vi "Test Null Assert.vi"(7 "Label (VI Title)":string, 8 "error in (no error)":errorcluster, 10 "Type in":variant, 11 "Type in":variant) -> (0 "error out":errorcluster)   [LabVIEW 2018, in "JSON to LVConstant Test.lvlib"]
uses:
  JSON to LVConstant Test.lvlib
  <vilib>/addons/_JKI Toolkits/Caraya/classes/Assert/Assert True.vi
  <vilib>/addons/_JKI Toolkits/Caraya/classes/Assert/Assert.lvclass
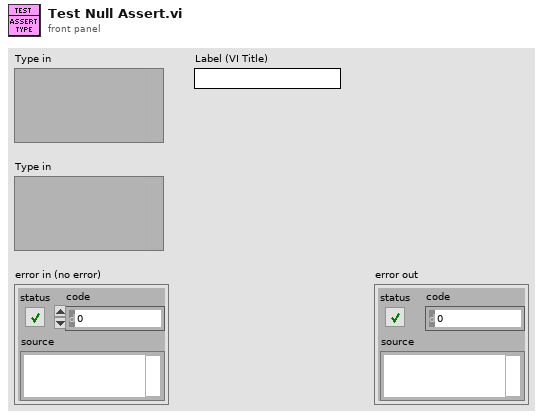
[diagram p1: front panel]
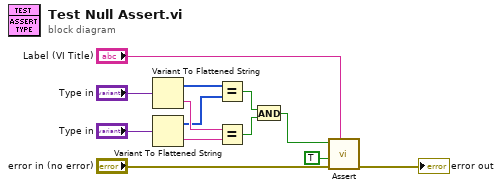
[diagram p0: block diagram]
diagram:
  n1 = Variant To Flattened String(Variant="Type in") -> (data string=w9:string, 1:w6:i16[])
  n2 = Variant To Flattened String(Variant="Type in") -> (data string=w8:string, 1:w7:i16[])
  n3 = Equal?(x=w6, y=w7) -> (x = y?=w11:bool)
  n4 = Equal?(x=w9, y=w8) -> (x = y?=w10:bool)
  n5 = And(x=w11, y=w10) -> (x .and. y?=w12:bool)
  n6 = call-poly <vilib>:"Assert.vi"("Label"="Label (VI Title)", "error in (no error)"="error in (no error)", "Register with caller test (F)"=TRUE, "True?"=w12) -> ("error out"=→"error out":errorcluster)  [unwired: 7 in]
